vi "Hardware Front Panel.vi"() -> ()   [LabVIEW 2009]
uses:
  <vilib>/userDefined/High Color/nirio_resource_hc.ctl
  <vilib>/rvi/interface/nirviOpenFPGA/nirviOpenFPGA.xnode
  FPGA Bitfiles/Q_IGVC_2010.lvproj_FPGA Target_FPGA_MAIN.vi.lvbitx
  <vilib>/rvi/errors/niLvFpgaWhatHappensToTopLevelVI.ctl
  <vilib>/rvi/interface/common/niFpgaNodeNameForErrorReporting.ctl
  <vilib>/rvi/errors/niLvFpgaAdjustHostInterfaceError.vi
  NiRioSrv.dll
  <vilib>/Utility/error.llb/Error Cluster From Error Code.vi
  <vilib>/rvi/interface/nirviMethod/nirviMethod.xnode
  <vilib>/rvi/interface/nirviReadWriteControl/nirviReadWriteControl.xnode
  <vilib>/rvi/interface/nirviCloseFPGA/nirviCloseFPGA.xnode
  FPGA/Control Panel/Hardware Control Panel States.ctl
  <vilib>/FPGAPlugInAG/cRIO-9113/nirviIntfOpen_cRIO-9113.vi
  <vilib>/Utility/error.llb/Merge Errors.vi
  <vilib>/LabVIEW Targets/FPGA/RIO/nirio_HostInterface/nirio_Reset.vi
  <vilib>/LabVIEW Targets/FPGA/RIO/nirio_HostInterface/nirio_DMAStopAll.vi
  <vilib>/LabVIEW Targets/FPGA/RIO/nirio_HostInterface/nirio_DisableInterrupts.vi
  <vilib>/RVI Host/nirviSupport.llb/nirviErrorClusterFromErrorCode.vi
  <vilib>/LabVIEW Targets/FPGA/RIO/nirio_HostInterface/nirio_EnableInterrupts.vi
  <vilib>/rvi/errors/niLvFpgaReportInternalErrorWithAdditionalInfo.vi
  <vilib>/FPGAPlugInAG/cRIO-9113/nirviIntfClose_cRIO-9113.vi
panel:
  out "HB LED ON/OFF/BLINK":u8
  out "Safety LED ON/OFF/BLINK":u8
  out "Init LED ON/OFF/BLINK":u8
  out "Current Control Panel State":T1=enum."Safety"
  in  "stop":bool
  out "Debounced Init Switch":bool
  out "Debounced Go Button":bool
  out "Debounced Safety Switch":bool
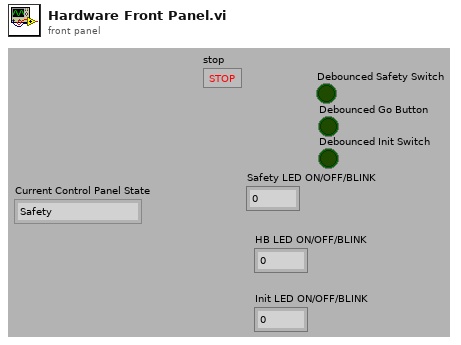
[diagram p1: front panel]
types:
  T1 = typedef "Hardware Control Panel States.ctl" = enum16{"Waiting for Init", "Init", "Waiting for Safety", "Safety", "Waiting for GO", "GO"}
  T2 = typedef "nirio_resource_hc.ctl" = tag
  T3 = typedef "niFpgaNodeNameForErrorReporting.ctl" = enum16{"Open FPGA VI Reference", "Read/Write Control", "Invoke Method: Abort", "Invoke Method: Acknowledge IRQ", "Invoke Method: Download", "Invoke Method: FIFO.Configure", "Invoke Method: FIFO.Read", "Invoke Method: FIFO.Start", "Invoke Method: FIFO.Stop", "Invoke Method: FIFO.Write", "Invoke Method: Reset", "Invoke Method: Run", "Invoke Method: Wait on IRQ", "Close FPGA VI Reference"}
  T4 = typedef "niLvFpgaWhatHappensToTopLevelVI.ctl" = enum16{"top level VI scripted behind XNode", "top level VI inlined behind XNode"}
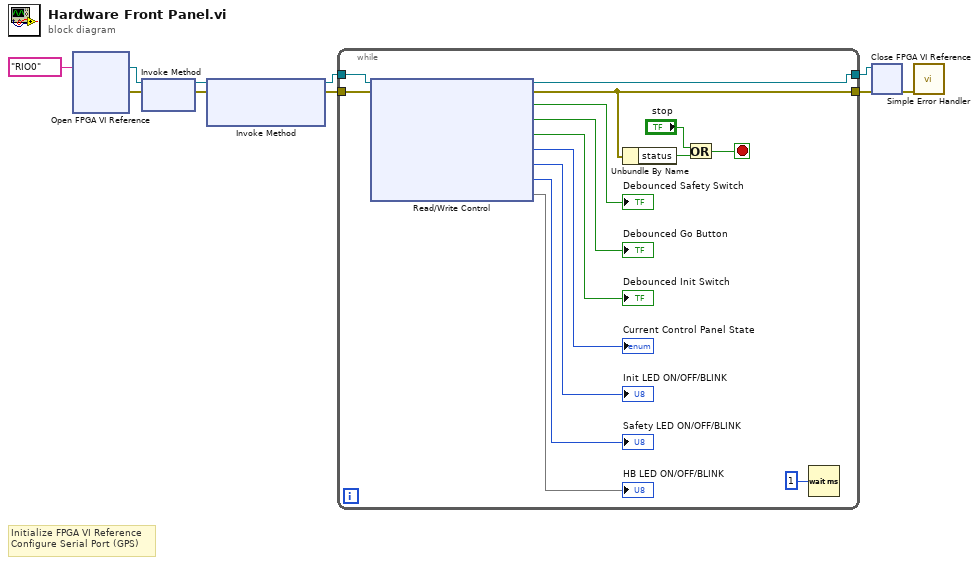
[diagram p0: block diagram]
diagram:
  # "Initialize FPGA VI Reference\nConfigure Serial Port (GPS)"
  n1 = xnode "Open FPGA VI Reference"("resource name"=T2 "RIO0") -> ("FPGA VI Reference Out"=w9:refnum<k20>, "error out"=w8:errorcluster)  [unwired: 1 in]
  n2 = xnode "Invoke Method"("FPGA VI Reference In"=w9, "error in"=w8) -> ("FPGA VI Reference Out"=w7:refnum<k20>, "error out"=w6:errorcluster)
  n3 = xnode "Invoke Method"("FPGA VI Reference In"=w7, "error in"=w6) -> ("FPGA VI Reference Out"=w5:refnum<k20>, "error out"=w4:errorcluster)  [unwired: 1 in]
  n4 = while {
    tunnel: w5 -> [w25]
    tunnel: w4 -> [w24]
    tunnel: [w20] -> w3
    tunnel: [w17] -> w2
    stop <- w18 stop-if-true
    n5 = xnode "Read/Write Control"("FPGA VI Reference In"=w25, "error in"=w24) -> ("FPGA VI Reference Out"=w20:refnum<k20>, "error out"=w17:errorcluster, "Debounced Safety Switch"=→"Debounced Safety Switch":bool, "Debounced Go Button"=→"Debounced Go Button":bool, "Debounced Init Switch"=→"Debounced Init Switch":bool, "Current Control Panel State"=→"Current Control Panel State":T1, "Init LED ON/OFF/BLINK"=→"Init LED ON/OFF/BLINK":u8, "Safety LED ON/OFF/BLINK"=→"Safety LED ON/OFF/BLINK":u8, "HB LED ON/OFF/BLINK"=→"HB LED ON/OFF/BLINK")
    n6 = Unbundle By Name(w17) -> ("status"=w16:bool)
    n7 = Or(x="stop", y=w16) -> (x .or. y?=w18:bool)
    n8 = Wait (ms)(milliseconds to wait=u32 1) -> ()  [unwired: 1 out]
  }
  n9 = xnode "Close FPGA VI Reference"("FPGA VI Reference In"=w3, "error in"=w2) -> ("error out"=w1:errorcluster)
  n10 = call <vilib>:"Simple Error Handler.vi"("error in (no error)"=w1) -> ()  [unwired: 4 in, 5 out]
